vi "relu_backward.vi"(1 "Z":dbl[][](array[numeric]), 2 "dA":dbl[][](array[numeric])) -> (0 "dZ":dbl[][](array[numeric]))   [LabVIEW 2020]
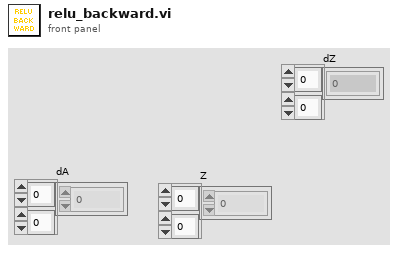
[diagram p1: front panel]
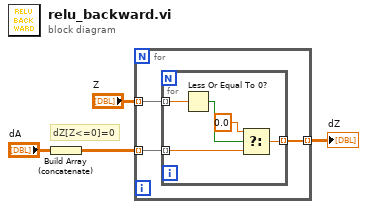
[diagram p0: block diagram]
diagram:
  # "dZ[Z<=0]=0"
  n1 = Build Array (concatenate)("dA") -> (w3:dbl[][])
  n2 = for {
    tunnel: w3 -> [w7] mode=indexing
    tunnel: "Z" -> [w6] mode=indexing
    tunnel: [w5] -> w1 mode=indexing
    n3 = for {
      tunnel: w7 -> [w9] mode=indexing
      tunnel: w6 -> [w12] mode=indexing
      tunnel: [w8] -> w5 mode=indexing
      n4 = Less Or Equal To 0?(x=w12) -> (x <= 0?=w11:bool)
      n5 = Select(t=0.0, s=w11, f=w9) -> (s? t:f=w8:dbl)
    }
  }
  "dZ" <- w1
